vi "Write Array.vi"(8 "error in (no error)":errorcluster, 9 "Data":u8[](array[numeric]), 10 "Timestamps":u64[](array[numeric]), 11 "Ring buffer DVR in":refnum<data-value>) -> (0 "error out":errorcluster, 3 "Ring buffer DVR out":refnum<data-value>)   [LabVIEW 2021, in "Ring Buffer Time Series Data.lvlib"]
uses:
  Ring Buffer Time Series Data.lvlib
  SubVIs/DVR data.ctl
  SubVIs/Enforce array size multiple timestamps.vi
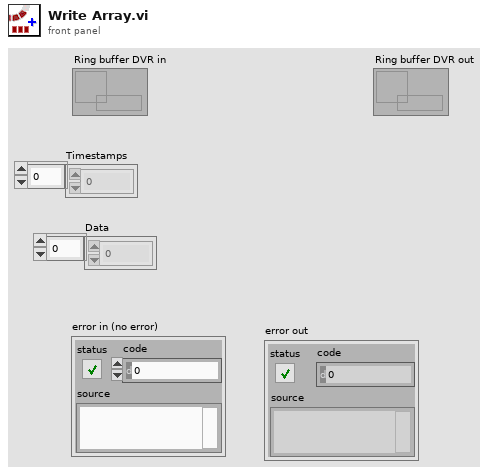
[diagram p1: front panel]
types:
  T1 = typedef "Ring Buffer Time Series Data.lvlib/DVR data.ctl" = cluster{"Timestamps":u64[], "Values":u8[], "#bytes per timestamp":i32, "Index":i32, "Size (#timestamps)":i32, "Full?":bool}
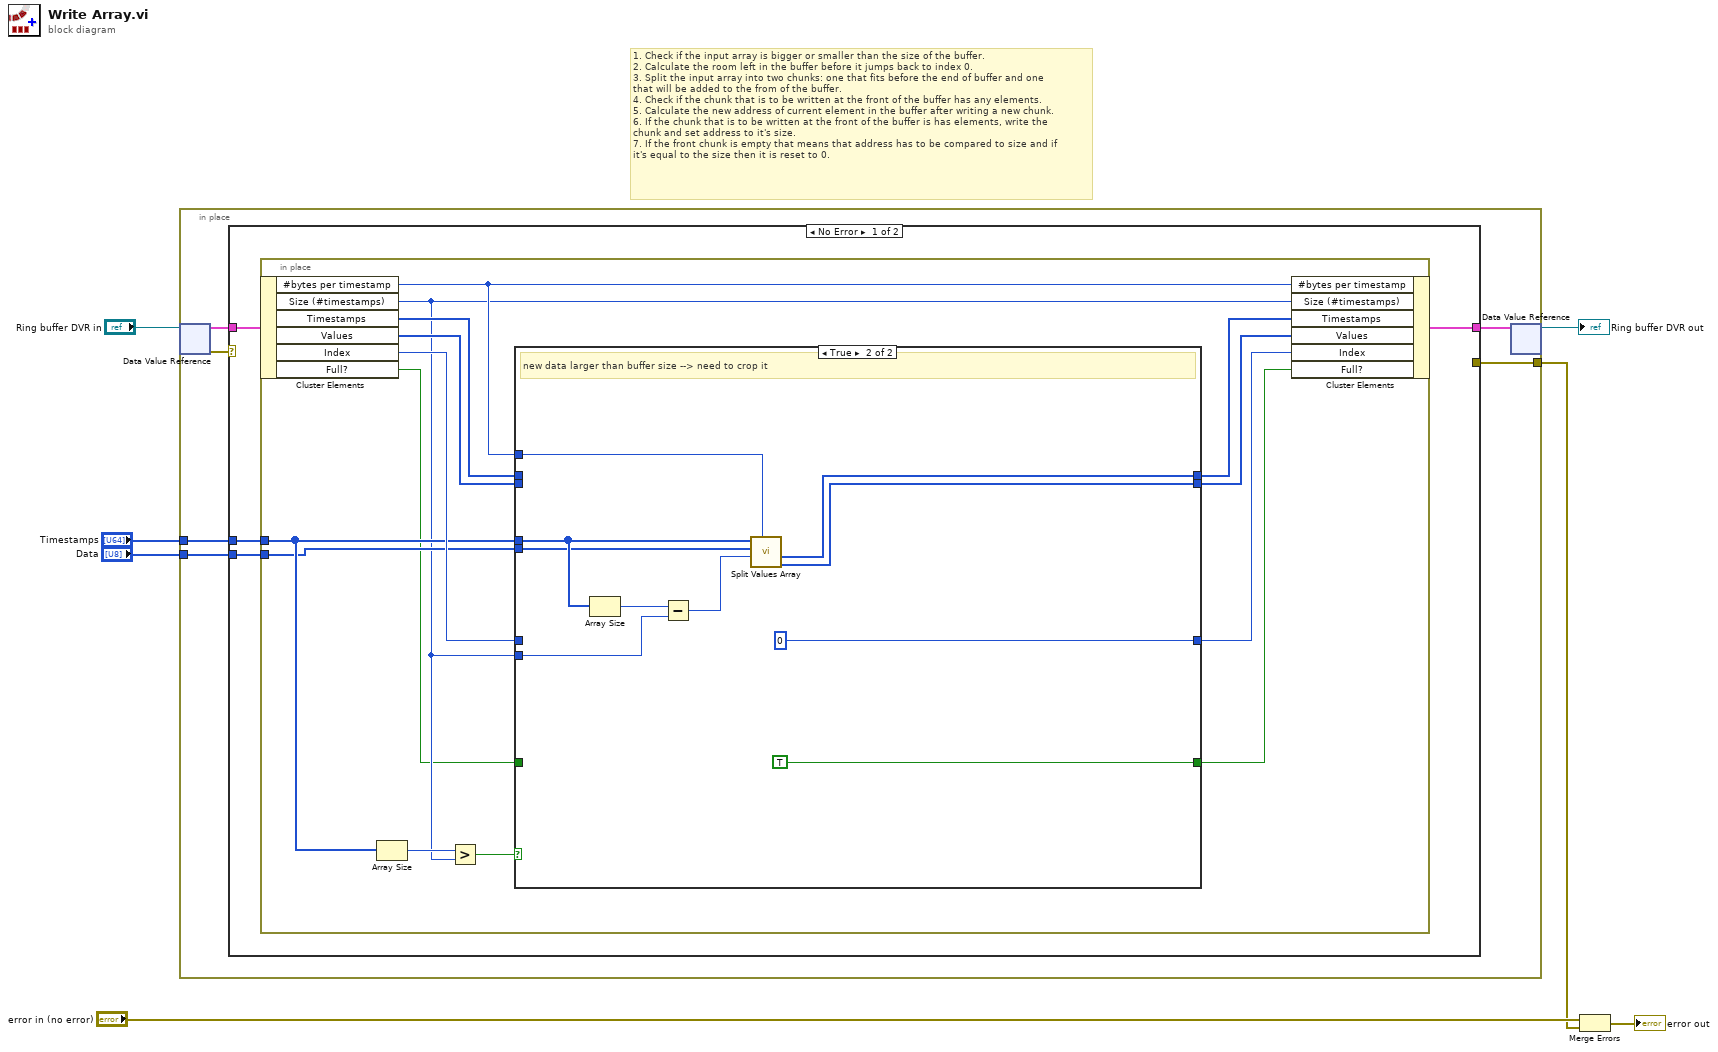
[diagram p0: block diagram]
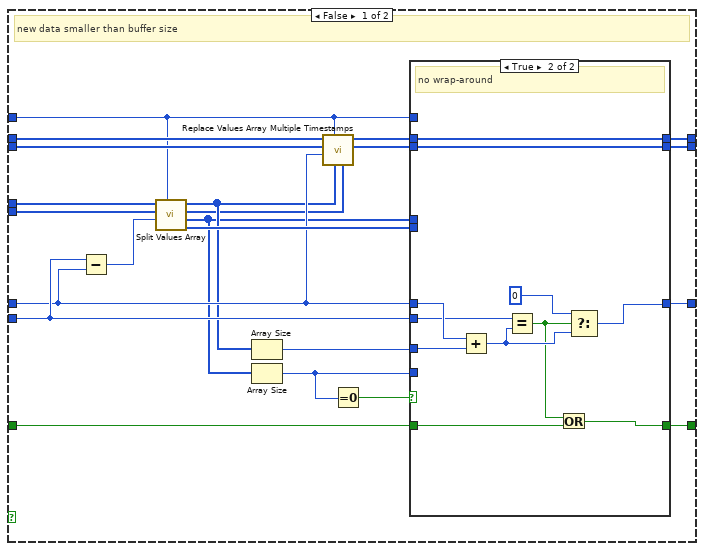
[diagram p2: hidden frame]
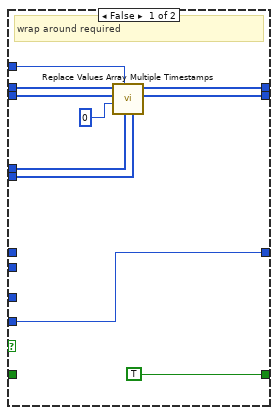
[diagram p3: hidden frame]
diagram:
  # "1. Check if the input array is bigger or smaller than the size of the buffer.\n2. Calculate the room left in the buffer before it jumps back to index 0.\n3. Split the input array into two chunks: one that fits before the end of buffer and one\nthat will be added to the from of the buffer.\n4. Check if the chunk that is to be written at the front of the buffer has any elements.\n5. Calculate the new address of current element in the buffer after writing a new chunk.\n6. If the chunk that is to be written at the front of the buffer is has elements, write the\nchunk and set address to it's size.\n7. If the front chunk is empty that means that address has to be compared to size and if\nit's equal to the size then it is reset to 0."
  n1 = in-place {
    in-place-border: [w10] -> w2
    in-place-border: "Timestamps" -> [w9]
    in-place-border: "Data" -> [w8]
    n2 = in-place-dvr #1("Ring buffer DVR in") -> (w12:T1, w13:errorcluster)
    n3 = case shown="No Error" w13 {
      selector: w13 -> [_ w85]
      tunnel: w12 -> [w17 _]
      tunnel: [w16 _] -> w11
      tunnel: [_ w85] -> w10
      tunnel: w9 -> [w15 _]
      tunnel: w8 -> [w14 _]
      frame No Error {
        n4 = in-place {
          in-place-border: w15 -> [w25]
          in-place-border: w14 -> [w24]
          n5 = in-place-cluster #2(w17) -> ("#bytes per timestamp"=w26:i32, "Size (#timestamps)"=w22:i32, "Timestamps"=w28:u64[], "Values"=w27:u8[], "Index"=w29:i32, "Full?"=w19:bool)
          n6 = Array Size(array=w25) -> (size(s)=w31:i32)
          n7 = Greater?(x=w31, y=w22) -> (0:w30:bool)
          n8 = case shown="True" w30 {
            tunnel: w22 -> [w46 w82]
            tunnel: w29 -> [w38 _]
            tunnel: w28 -> [w40 _]
            tunnel: w27 -> [w39 _]
            tunnel: w26 -> [w33 w79]
            tunnel: w25 -> [w51 w83]
            tunnel: w24 -> [w50 w80]
            tunnel: [w45 0 ("t")] -> w23
            tunnel: [w44 w78] -> w21
            tunnel: [w43 w77] -> w20
            tunnel: w19 -> [w42 _]
            tunnel: [w41 TRUE] -> w18
            frame False {
              # "new data smaller than buffer size"
              n9 = Subtract(x=w46, y=w38) -> (x-y=w53:i32)
              n10 = call "Split Values Array.vi"("#bytes per timestamp"=w33, "split index"=w53, "Values"=w50, "Timestamps"=w51) -> ("Values (post-split)"=w49:u8[], "Timestamps (post-split)"=w32:u64[], "Values (pre-split)"=w36:u8[], "Timestamps (pre-split)"=w37:u64[])  [unwired: 4 in]
              n11 = Array Size(array=w37) -> (size(s)=w47:i32)
              n12 = Array Size(array=w32) -> (size(s)=w48:i32)
              n13 = call "Replace Values Array Multiple Timestamps.vi"("Values (new)"=w36, "Timestamps (new)"=w37, "#bytes per timestamp"=w33, "index"=w38, "Values (buffered)"=w39, "Timestamps (buffered)"=w40) -> ("Values (buffered)"=w34:u8[], "Timestamps (buffered)"=w35:u64[])  [unwired: 4 in]
              n14 = Equal To 0?(x=w48) -> (x = 0?=w52:bool)
              n15 = case shown="True" w52 {
                tunnel: w35 -> [w61 w68]
                tunnel: w34 -> [w60 w67]
                tunnel: w33 -> [w57 _]
                tunnel: w32 -> [w56 _]
                tunnel: w49 -> [w55 _]
                tunnel: w38 -> [_ w73]
                tunnel: w48 -> [w63 _]
                tunnel: w47 -> [_ w72]
                tunnel: w46 -> [_ w70]
                tunnel: [w63 w69] -> w45
                tunnel: [w59 w68] -> w44
                tunnel: [w58 w67] -> w43
                tunnel: w42 -> [_ w66]
                tunnel: [TRUE w64] -> w41
                frame False {
                  # "wrap around required"
                  n16 = call "Replace Values Array Multiple Timestamps.vi"("Values (new)"=w55, "Timestamps (new)"=w56, "#bytes per timestamp"=w57, "index"=0, "Values (buffered)"=w60, "Timestamps (buffered)"=w61) -> ("Values (buffered)"=w58:u8[], "Timestamps (buffered)"=w59:u64[])  [unwired: 4 in]
                }
                frame True {
                  # "no wrap-around"
                  n17 = Add(x=w73, y=w72) -> (x+y=w71:i32)
                  n18 = Equal?(x=w70, y=w71) -> (x = y?=w65:bool)
                  n19 = Or(x=w65, y=w66) -> (x .or. y?=w64:bool)
                  n20 = Select(t=0, s=w65, f=w71) -> (s? t:f=w69:i32)
                }
              }
            }
            frame True {
              # "new data larger than buffer size --> need to crop it"
              n21 = Array Size(array=w83) -> (size(s)=w84:i32)
              n22 = Subtract(x=w84, y=w82) -> (x-y=w81:i32)
              n23 = call "Split Values Array.vi"("#bytes per timestamp"=w79, "split index"=w81, "Values"=w80, "Timestamps"=w83) -> ("Values (post-split)"=w77:u8[], "Timestamps (post-split)"=w78:u64[])  [unwired: 4 in, 2 out]
            }
          }
          n24 = in-place-cluster #2("#bytes per timestamp"=w26, "Size (#timestamps)"=w22, "Timestamps"=w21, "Values"=w20, "Index"=w23, "Full?"=w18) -> (w16:T1)
        }
      }
      frame Error {
      }
    }
    n25 = in-place-dvr #1(w11) -> (→"Ring buffer DVR out":refnum<data-value>)  [unwired: 1 out]
  }
  n26 = Merge Errors("error in (no error)", w2) -> (→"error out":errorcluster)
